vi "read-PLT-corel.vi"(5 "file (use dialog)":path) -> (0 "Y":ext[](array[numeric]), 1 "Pen":bool[](array[boolean]), 2 "X":ext[](array[numeric]))   [LabVIEW 2014]
doc: "André Romero - 2016\nandretec@ifsc.usp.br\n\nRead PLT files and convert in coordenates"
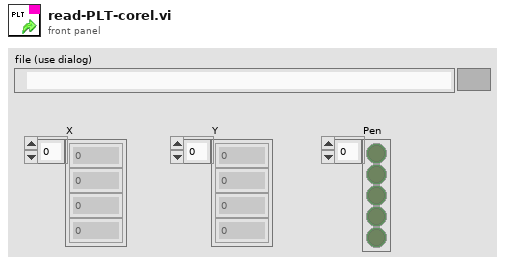
[diagram p1: front panel]
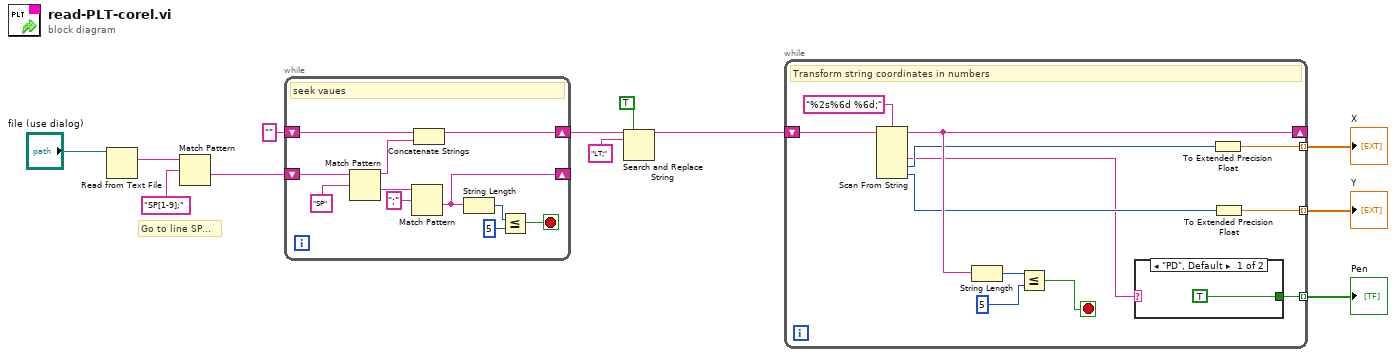
[diagram p0: block diagram]
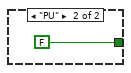
[diagram p2: hidden frame]
diagram:
  # "Go to line SP..."
  n1 = Read from Text File(file (use dialog)="file (use dialog)") -> (text=w12:string)  [unwired: 3 in, 3 out]
  n2 = Match Pattern(string=w12, regular expression="SP[1-9];") -> (after substring=w2:string)  [unwired: 1 in, 3 out]
  n3 = while {
    shift-right: [w17] -> _
    shift-left: w2 -> [w20]
    shift-right: [w18] -> w3
    shift-left: "" -> [w19]
    stop <- w14 stop-if-true
    # "seek vaues"
    n4 = Match Pattern(string=w20, regular expression="SP" ("search string")) -> (before substring=w13:string, after substring=w22:string)  [unwired: 1 in, 2 out]
    n5 = Match Pattern(string=w22, regular expression=";") -> (after substring=w17:string)  [unwired: 1 in, 3 out]
    n6 = Concatenate Strings(w19, w13) -> (w18:string)
    n7 = String Length(string=w17) -> (length=w16:i32)
    n8 = Less Or Equal?(x=w16, y=5) -> (x <= y?=w14:bool)
  }
  n9 = Search and Replace String(replace all?=TRUE ("replace all? (F)"), input string=w3, search string="LT;") -> (result string=w1:string)  [unwired: 5 in, 3 out]
  n10 = while {
    shift-right: [w33] -> _
    shift-left: w1 -> [w34]
    tunnel: [w25] -> w6 mode=indexing
    tunnel: [w24] -> w5 mode=indexing
    tunnel: [w26] -> w4 mode=indexing
    stop <- w30 stop-if-true
    # "Transform string coordinates in numbers"
    n11 = Scan From String(format string="%2s%6d %6d;", input string=w34) -> (remaining string=w33:string, output 1=w27:string, output 2=w29:i32, output 3=w28:i32)  [unwired: 5 in, 2 out]
    n12 = String Length(string=w33) -> (length=w32:i32)
    n13 = Less Or Equal?(x=w32, y=5) -> (x <= y?=w30:bool)
    n14 = case shown="\"PD\", Default" w27 {
      tunnel: [TRUE FALSE] -> w26
      frame "PD", Default {
      }
      frame "PU" {
      }
    }
    n15 = To Extended Precision Float(1:w29) -> (0:w25:ext)
    n16 = To Extended Precision Float(1:w28) -> (0:w24:ext)
  }
  "X" <- w6
  "Y" <- w5
  "Pen" <- w4
